vi "Pfeiffer Vacuum OnTool Monitoring Operating Pumpsys.vi"(8 "error in (no error)":errorcluster, 9 "PV OnTool Monitoring Op - Cluster":T1={"Parameter"=0, "Parameter\nread only<->describe"=FALSE, "Softpumping\nswitching\nthreshhold [hPa]"=267, "Soft pump rotation\nspeed in % of the\nfinal rpm [%]"=15, "Lower exhaust\ngas temperature\nlimit [C] "=5, "Upper exhaust\ngas temperature\nlimit [C]  "=250, "End of measuring\nrange of gauge"=0} {"End of measuring\nrange of gauge" items=[" 10 hPa", " 100 hPa", " 1000 hPa"]; "Upper exhaust\ngas temperature\nlimit [C]" min=5 max=250 step=1; "Lower exhaust\ngas temperature\nlimit [C]" min=5 max=200 step=1; "Soft pump rotation\nspeed in % of the\nfinal rpm [%]" min=15 max=100 step=1; "Softpumping\nswitching\nthreshhold [hPa]" min=0 max=1000 step=1; "Parameter" items=[" End of measuring range of gauge", " Exhaust pressure  [h/Pa]  (read only)", " Intake pressure  [hPa]  (read only)", " Temperature of pump housing [°C]   (read only)", " Motor temperature pump [°C] (read only)", " Temperature of exhaust gas [°C]   (read only)", " Softpumping switching threshhold [hPa]", " Soft pump rotation speed in % of the final rpm [%]", " Lower exhaust gas temperature limit [C]  ", " Upper exhaust gas temperature limit [C] "]}, 10 "Adress of unit":u16=1 min=1 max=999 step=1, 11 "COM Port Name in":refnum<visa-resource-name>="COM1") -> (0 "error out":errorcluster, 1 "response (data)":string)   [LabVIEW 2016]
doc: "This VI is an example of how to use the Pfeiffer Vacuum subVIs programmatically. This VI first initializes the instrument, takes measurements, then closes the instrument."
uses:
  Public/OnTool/PV OnTool Monitoring Op - Cluster.ctl
  Pfeiffer Vacuum.lvlib
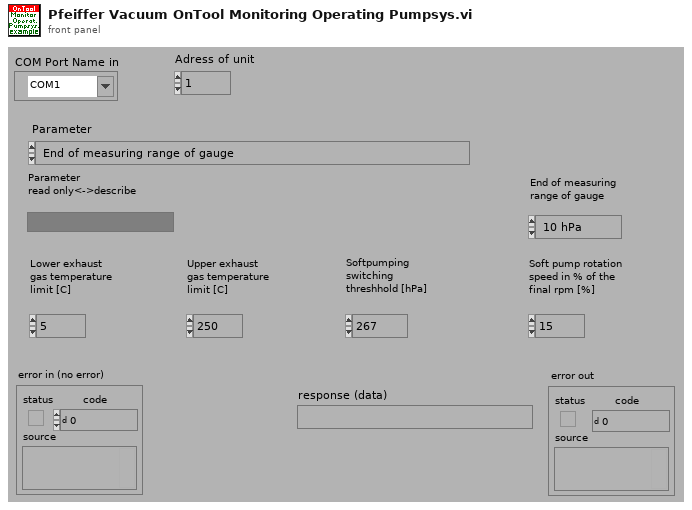
[diagram p1: front panel]
types:
  T1 = typedef "Pfeiffer Vacuum.lvlib/PV OnTool Monitoring Op - Cluster.ctl" = cluster{"Parameter":u16, "Parameter\nread only<->describe":bool, "Softpumping\nswitching\nthreshhold [hPa]":i16, "Soft pump rotation\nspeed in % of the\nfinal rpm [%]":u16, "Lower exhaust\ngas temperature\nlimit [C] ":u16, "Upper exhaust\ngas temperature\nlimit [C]  ":u16, "End of measuring\nrange of gauge":u16}
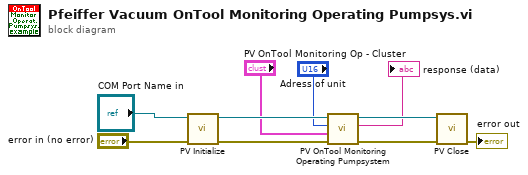
[diagram p0: block diagram]
diagram:
  n1 = call "PV Initialize.vi"("error in (no error)"="error in (no error)", "VISA session in"="COM Port Name in") -> ("error out"=w8:errorcluster, "VISA session out"=w6:refnum<visa-resource-name>)  [unwired: 8 in]
  n2 = call "PV OnTool Monitoring Operating Pumpsystem.vi"("error in (no error)"=w8, "PV OnTool Monitoring Op - Cluster"="PV OnTool Monitoring Op - Cluster", "Adress of unit"="Adress of unit", "VISA session"=w6) -> ("error out"=w7:errorcluster, "response (data)"=→"response (data)":string, "dup VISA session"=w5:refnum<visa-resource-name>)  [unwired: 5 in]
  n3 = call "PV Close.vi"("VISA session"=w5, "error in (no error)"=w7) -> ("error out"=→"error out":errorcluster)  [unwired: 13 in]
